vi "LCP Create Conti Flow Pump.vi"(8 "error in (no error)":errorcluster caption="Fehler (Eingang, kein Fehler)", 10 "SyringePump2":i64, 11 "SyringePump1":i64) -> (0 "error out":errorcluster caption="Fehler (Ausgang)", 3 "ContiFlowPumpHandle":i64)   [LabVIEW 2021, in "labbCAN_Pump_API.lvlib"]
uses:
  labbCAN_Pump_API.lvlib
  labbCAN_Pump_API.dll
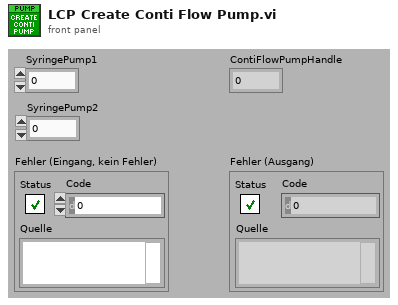
[diagram p1: front panel]
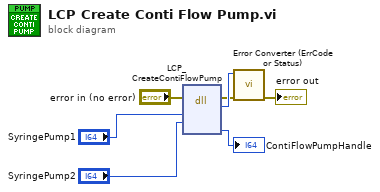
[diagram p0: block diagram]
diagram:
  n1 = dll-call lib="C:/Users/olaja/AppData/Local/CETONI_SDK/labbCAN_Pump_API.*" fn="LCP_CreateContiFlowPump"(error in="error in (no error)", "hPump1"="SyringePump1", "hPump2"="SyringePump2") -> (error out=w4:errorcluster, "Rückgabetyp"=w7:i32, "ContiFlowPumpHandle"=→"ContiFlowPumpHandle":i64)  [unwired: 5 in, 1 out]
  n2 = call "Error Converter (ErrCode or Status).vi"("error in (no error)"=w4, "error code"=w7) -> ("error out"=→"error out":errorcluster)  [unwired: 9 in]
